vi "Set Data.vi"(8 "error in":errorcluster, 10 "DataIn":sgl[](array[numeric]), 11 "AlicatMData in":refnum<class "AlicatMCData.lvclass">) -> (0 "error out":errorcluster, 3 "AlicatMData out":refnum<class "AlicatMCData.lvclass">)   [LabVIEW 2015, in "Alicat.lvlib" / "AlicatMCData.lvclass"]
uses:
  AlicatMCData.lvclass
  AlicatMCData.lvclass/AlicatMCData.ctl
  Reusable/General/Atmospheric/Atmospheric Constants.vi
  Reusable/General/Atmospheric/Atmospheric Library.lvlib
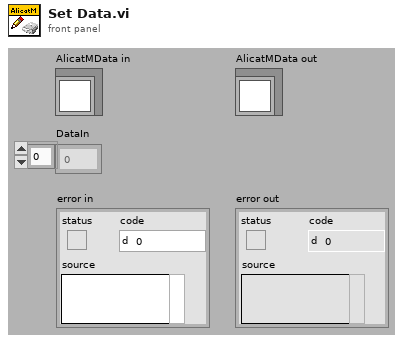
[diagram p1: front panel]
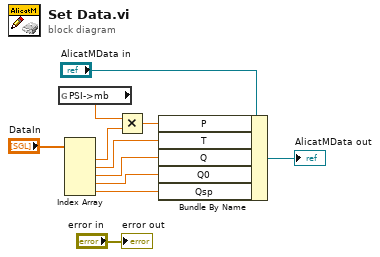
[diagram p0: block diagram]
diagram:
  n1 = global read "Atmospheric Constants.vi" "PSI->mb"() -> (w1:sgl)
  n2 = Index Array(array="DataIn") -> (element #1=w6:sgl, element #2=w5:sgl, element #3=w4:sgl, element #4=w3:sgl, element #5=w2:sgl)  [unwired: 5 in]
  n3 = Multiply(x=w1, y=w6) -> (x*y=w7:sgl)
  n4 = Bundle By Name(cluster="AlicatMData in", "P"=w7, "T"=w5, "Q"=w4, "Q0"=w3, "Qsp"=w2) -> (→"AlicatMData out":refnum<class "AlicatMCData.lvclass">)
  "error out" <- "error in"
